vi "Consumer.vi"(8 "error in (no error)":errorcluster, 9 "Data":variant, 10 "Case ID":string, 11 "uService Template in":refnum<class "Common GUI v3.lvclass">) -> (0 "error out":errorcluster, 3 "uService Template out":refnum<class "Common GUI v3.lvclass">)   [LabVIEW 2026, in "TALOS.lvlib" / "Common GUI v3.lvlib" / "Common GUI v3.lvclass"]
uses:
  Common GUI v3.lvclass
  C:/LabVIEW Code/TALOS/talos/Ancestor/Ancestor/Ancestor.lvclass
  Common GUI v3 Consumer Case Selector.ctl
  Classes/Guardian List/Guardian List.lvclass
  Common GUI v3.lvclass/Common GUI v3.ctl
  Ancestor/Ancestor/Ancestor.lvclass/Ancestor.ctl
  Error Listbox Msg.ctl
  Error Listbox Msg Action.ctl
  Error Manager/Error Info.ctl
  Remote uService GUI.ctl
  Classes/uService List/uService List.lvclass/uService List.ctl
  Classes/uService List/Get Remote GUI.vi
  Classes/uService List/Get Remote Window VI Ref.vi
  Classes/uService List/Set Remote Window VI Ref.vi
  Classes/uService List/Get VI Ref.vi
  Support VIs/Generate Error.vi
  FGV/Error Memory/Get Error Description.vi
  Support VIs/Get PC name.vi
  Ancestor/Ancestor/Read ID.vi
  Support VIs/Get Class Name.vi
  FGV/Error Memory/Error Memory Core.vi
  <vilib>/AdvancedString/Delimited String to 1D String Array.vi
  <vilib>/AdvancedString/Delimited String to 1D String Array (string).vi
  Support VIs/Circus Root Path.vi
  FGV/Error Memory/Error Crt Lvl checker.vi
  FGV/Error Memory/Error Memory Core.vi/40c8088d-b597-4017-91af-faa98e00292e.vi
  FGV/Error Memory/Error Memory Core.vi/d4a3ab98-063c-4e44-b43d-fbdcfe6c2be2.vi
  Support VIs/Global Memory.vi
  <vilib>/Utility/LVClass/Get LV Class Name.vi
  Support VIs/Is in Packed Library.vi
  Support VIs/TALOS Root path.vi
  Support VIs/Read CSV worksheet.vi
  Support VIs/Global Constants.vi
  <vilib>/Utility/error.llb/General Error Handler.vi
  Support VIs/Error Log.vi
  Ancestor/Ancestor/Ancestor.lvclass
  <vilib>/Comparison/Equal/Equal Functor/Equal Functor.lvclass
  Classes/uService List/uService List.lvclass
  Father of all uServices/Father of all uServices/Father of all uServices.lvclass
  TALOS.lvlib
  Error Manager/Error Manager.lvclass
  Common GUI v3.lvlib
  Guardian/Guardian/Guardian.lvclass
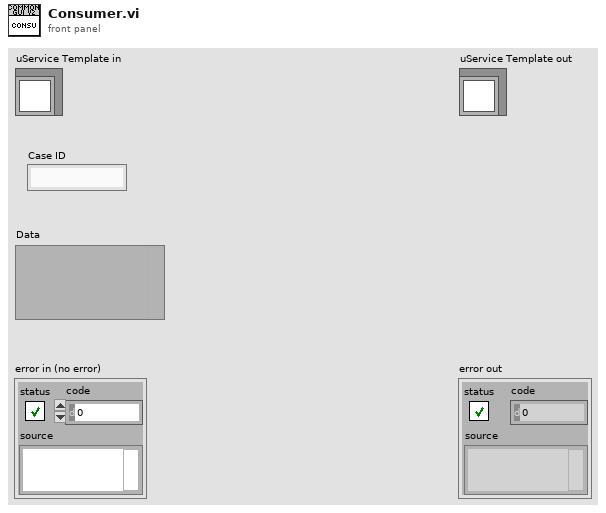
[diagram p1: front panel]
types:
  T1 = typedef "TALOS.lvlib/Common GUI v3.lvlib/Common GUI v3.lvclass/Common GUI v3 Consumer Case Selector.ctl" = enum16{"Update Guardians List", "Update ABORT LED", "Update Guardian ID", "Update Kasli Log", "Update Error Listbox", "Update Run Number", "Change Run LED color", "Update Run Status", "Run Stopped with Errors", "Reset Run LED", "Update Run Config", "Remote GUI"}
  T2 = typedef "TALOS.lvlib/Common GUI v3.lvlib/Common GUI v3.lvclass/Error Listbox Msg.ctl" = cluster{"Action":T3, "Error Info":T4}
  T3 = typedef "TALOS.lvlib/Common GUI v3.lvlib/Common GUI v3.lvclass/Error Listbox Msg Action.ctl" = enum16{"Add", "Remove", "Clear"}
  T4 = typedef "TALOS.lvlib/Error Manager.lvlib/Error Manager.lvclass/Error Info.ctl" = cluster{"error out":errorcluster, "Time Stamp":timestamp, "Machine Name":string, "GUID":string}
  T5 = typedef "TALOS.lvlib/Common GUI v3.lvlib/Remote uService GUI.ctl" = cluster{"Open/Close":bool, "uService ID":string}
  T6 = map{string, cluster{"Online":bool, "Last Poke":timestamp}}
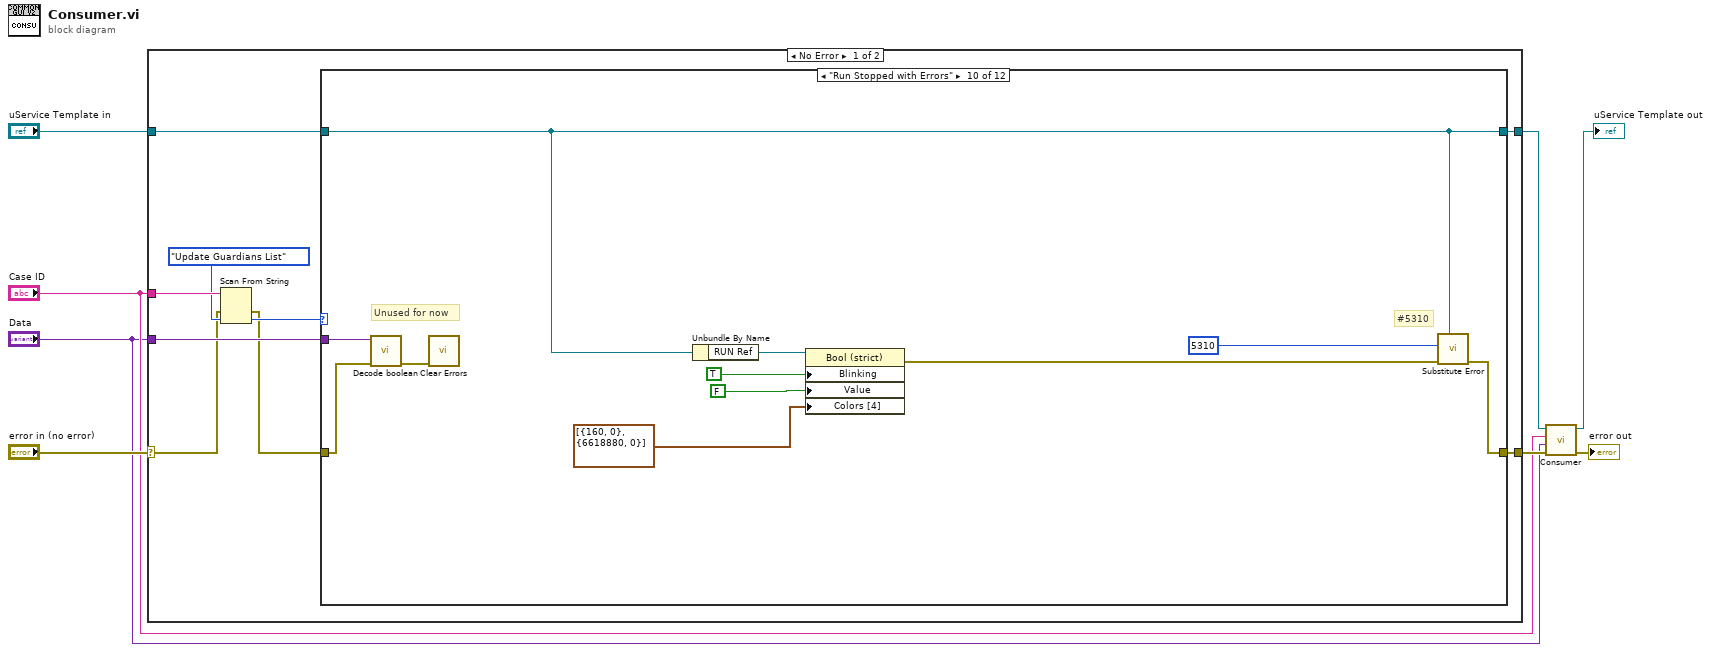
[diagram p0: block diagram]
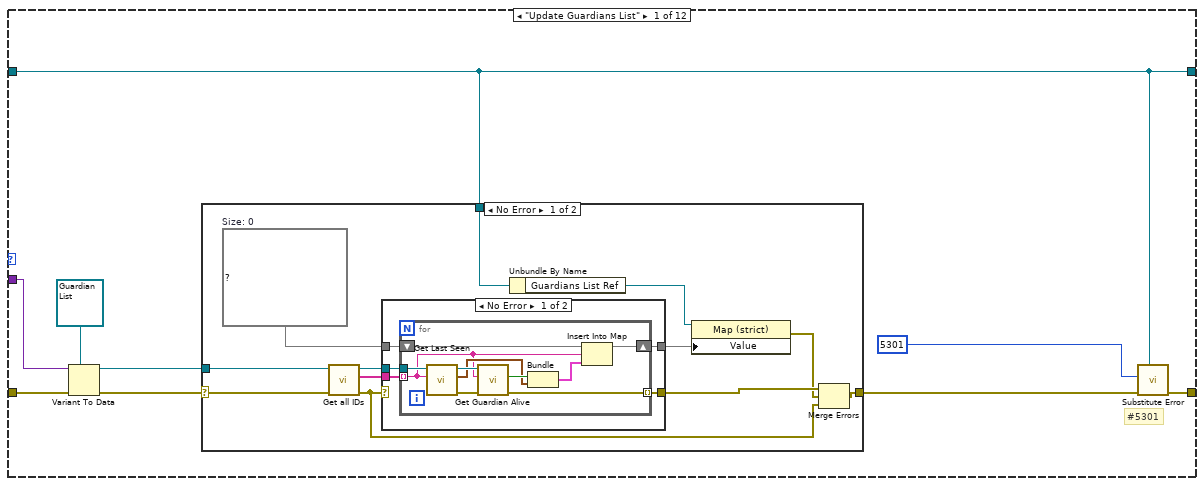
[diagram p2: hidden frame]
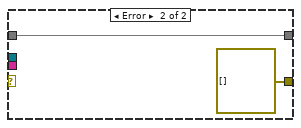
[diagram p3: hidden frame]
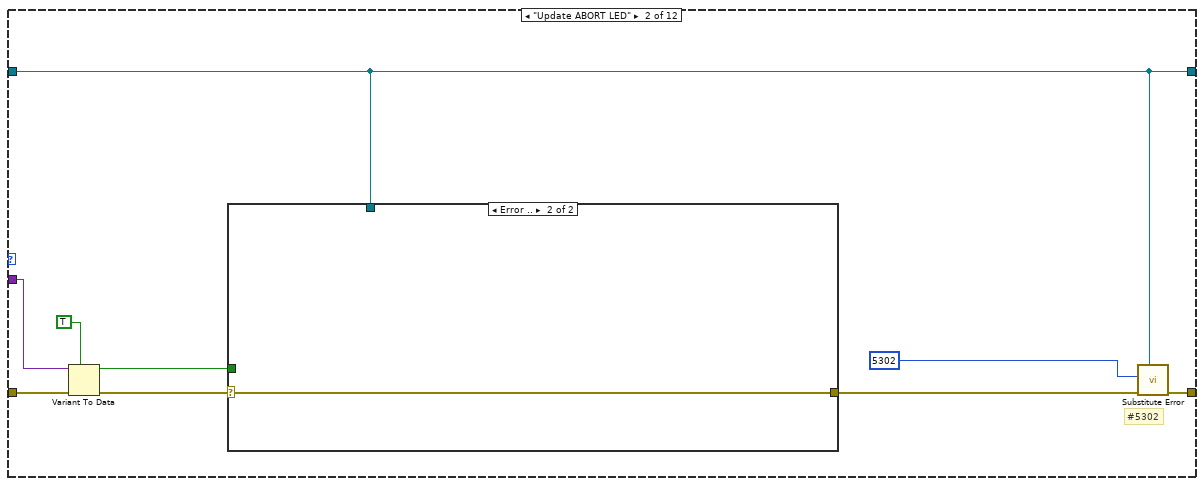
[diagram p5: hidden frame]
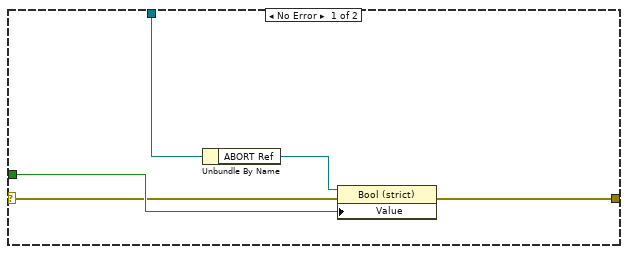
[diagram p6: hidden frame]
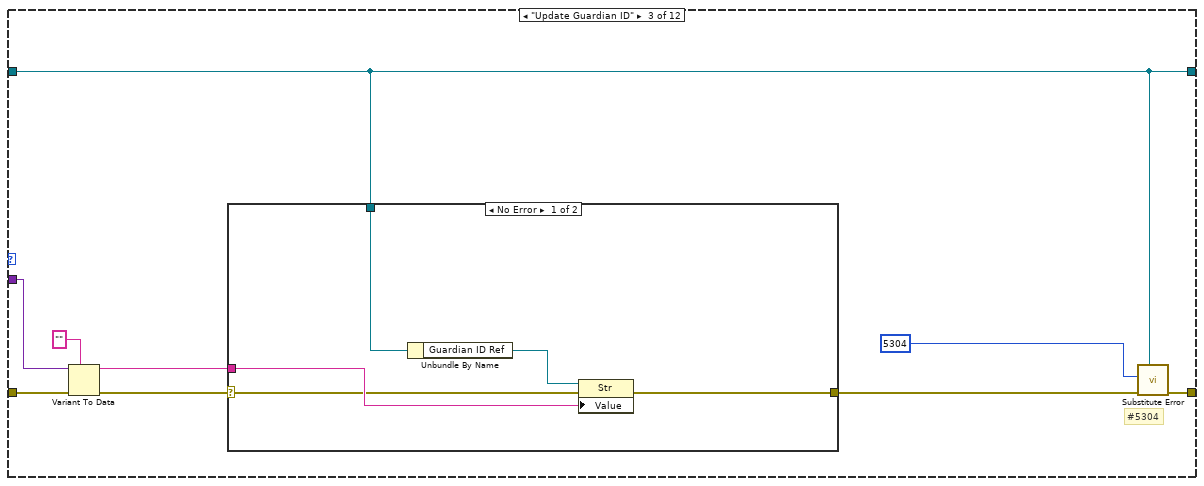
[diagram p7: hidden frame]
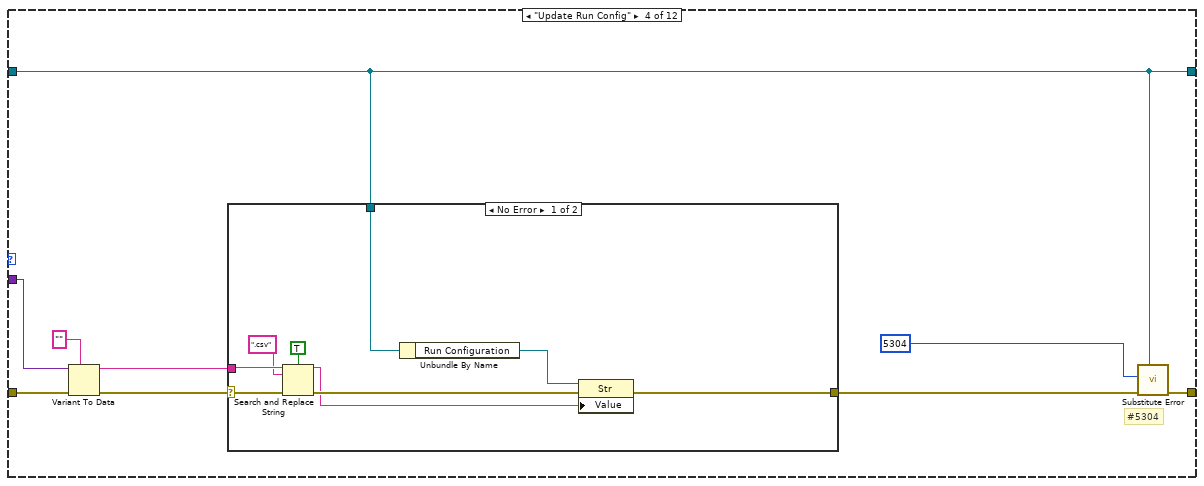
[diagram p9: hidden frame]
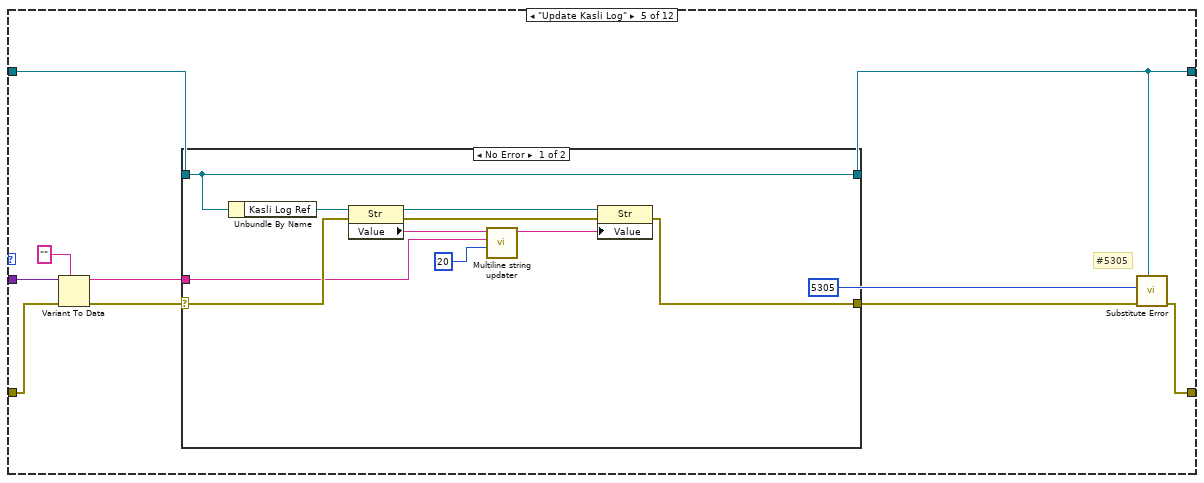
[diagram p11: hidden frame]
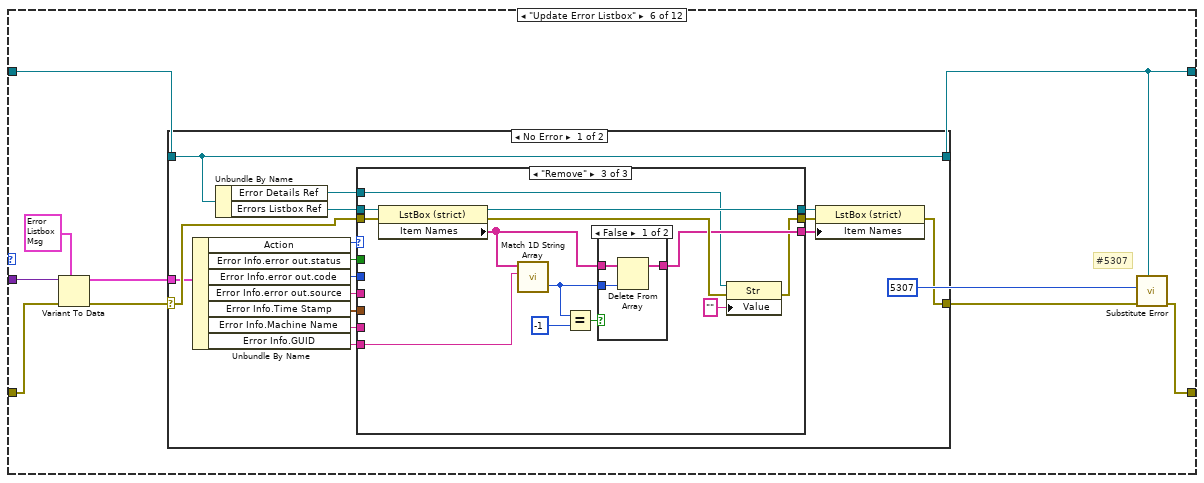
[diagram p13: hidden frame]
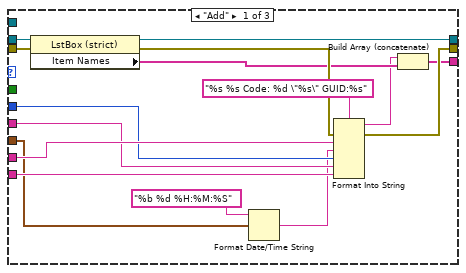
[diagram p14: hidden frame]
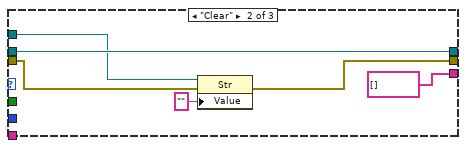
[diagram p15: hidden frame]
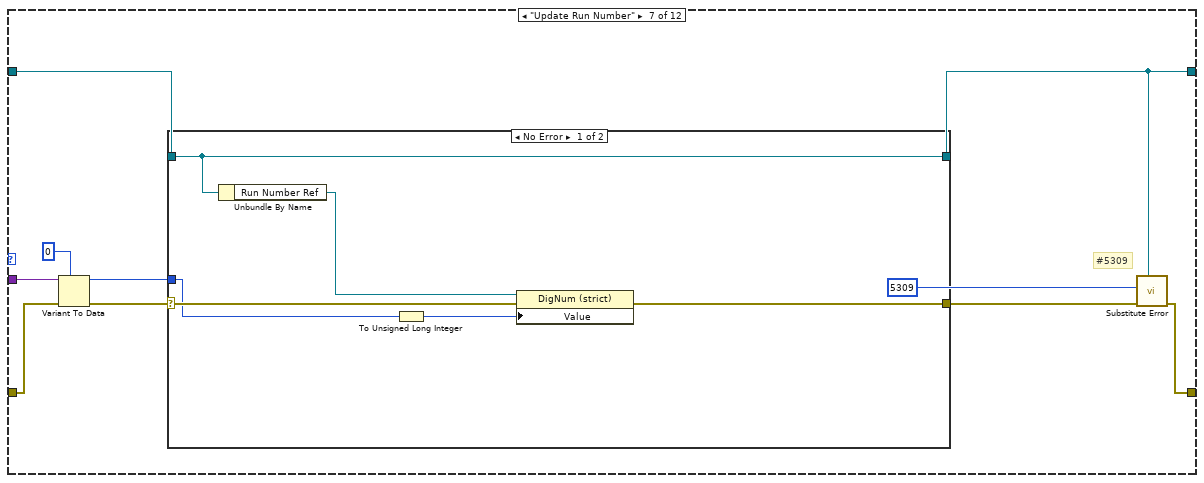
[diagram p18: hidden frame]
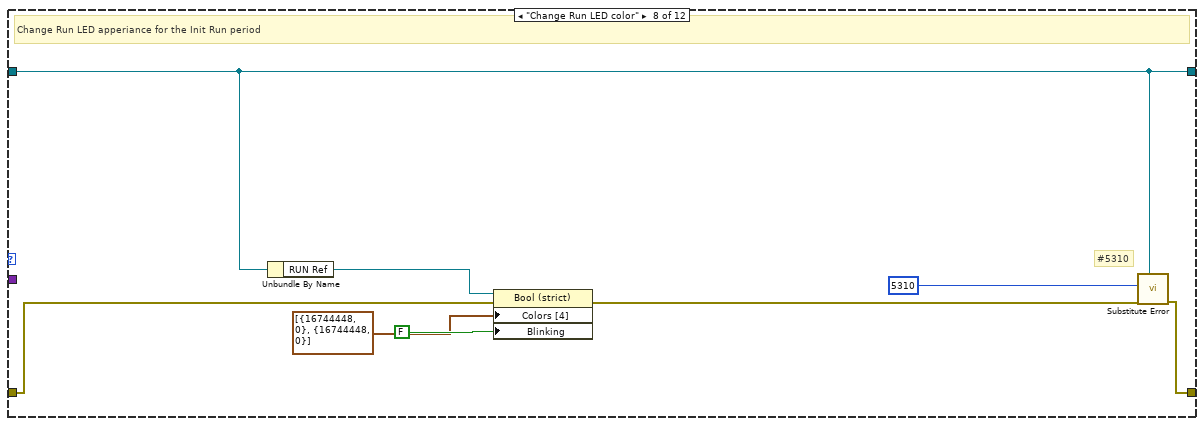
[diagram p20: hidden frame]
diagram:
  n1 = case shown="No Error" "error in (no error)" {
    selector: "error in (no error)" -> [w10 w352]
    tunnel: "uService Template in" -> [w16 w353]
    tunnel: [w14 w353] -> w4
    tunnel: [w15 w352] -> w3
    tunnel: "Case ID" -> [w13 _]
    tunnel: "Data" -> [w17 _]
    frame No Error {
      n2 = Scan From String(input string=w13, error in=w10, default 1=Common_GUI_v3_Consumer_Case_Selector."Update Guardians List") -> (error out=w9:errorcluster, output 1=w11:T1)  [unwired: 2 in, 2 out]
      n3 = case shown="\"Run Stopped with Errors\"" w11 {
        tunnel: w17 -> [w23 w63 w78 w93 w114 w136 w203 _ w225 w239 _ w260]
        tunnel: w9 -> [w22 w62 w77 w92 w112 w135 w202 w216 w224 w238 _ w259]
        tunnel: w16 -> [w19 w59 w74 w89 w115 w137 w204 w217 w226 w243 w249 w257]
        tunnel: [w20 w60 w75 w90 w109 w132 w199 w218 w227 w244 w250 w258] -> w15
        tunnel: [w19 w59 w74 w89 w108 w131 w198 w217 w226 w243 w249 w255] -> w14
        frame "Update Guardians List" {
          # "#5301"
          n4 = Variant To Data(error in=w22, type=refnum<class "Guardian List.lvclass"> refnum ("Guardian List in"), Variant=w23) -> (data=w24:refnum<class "Guardian List.lvclass">, error out=w26:errorcluster)
          n5 = case shown="No Error" w26 {
            selector: w26 -> [w35 w56]
            tunnel: w24 -> [w34 _]
            tunnel: w19 -> [w32 _]
            tunnel: [w29 w56] -> w21
            frame No Error {
              w36 = T6 {}  # Size: 0
              n6 = call-dynamic "Get all IDs.vi"("error in (no error)"=w35, "Guardian List in"=w34) -> ("error out"=w27:errorcluster, "All IDs"=w38:string[], "Guardian List out"=w37:refnum<class "Guardian List.lvclass">)  [unwired: 7 in]
              n7 = case shown="No Error" w27 {
                tunnel: w38 -> [w43 _]
                tunnel: w37 -> [w42 _]
                tunnel: w36 -> [w41 w55]
                tunnel: [w40 errorcluster[] []] -> w33
                tunnel: [w39 w55] -> w30
                frame No Error {
                  n8 = for {
                    tunnel: w43 -> [w47] mode=indexing
                    tunnel: w42 -> [w53]
                    shift-right: [w48] -> w39
                    shift-left: w41 -> [w49]
                    tunnel: [w45] -> w40 mode=indexing
                    n9 = call-dynamic "Get Last Seen.vi"("ID"=w47, "Guardian List in"=w53) -> ("error out"=w44:errorcluster, "Last Poke"=w50:timestamp, "Guardian List out"=w52:refnum<class "Guardian List.lvclass">)  [unwired: 7 in]
                    n10 = call-dynamic "Get Guardian Alive.vi"("error in (no error)"=w44, "ID"=w47, "Guardian List in"=w52) -> ("error out"=w45:errorcluster, "Alive"=w51:bool)  [unwired: 6 in, 1 out]
                    n11 = Bundle("Alive"=w51, "Last Poke"=w50) -> (w46:cluster{"Alive":bool, "Last Poke":timestamp})  [unwired: 1 in]
                    n12 = Insert Into Map(map in=w49, key=w47, value=w46) -> (map out=w48:T6)  [unwired: 2 out]
                  }
                }
                frame Error {
                }
              }
              n13 = Unbundle By Name(w32) -> ("Guardians List Ref"=w31:refnum<vi>)
              n14 = property class="Map (strict)"(reference=w31, "Value"=w30) -> (error out=w28:errorcluster)  [unwired: 1 in, 1 out]
              n15 = Merge Errors(w33, w28, w27) -> (w29:errorcluster)
            }
            frame Error {
            }
          }
          n16 = call "Substitute Error.vi"("LabVIEW Object"=w19, "error in (no error)"=w21, "Error Code"=5301) -> ("error out"=w20:errorcluster)  [unwired: 8 in]
        }
        frame "Update ABORT LED" {
          # "#5302"
          n17 = Variant To Data(error in=w62, type=TRUE, Variant=w63) -> (data=w64:bool, error out=w65:errorcluster)
          n18 = case shown="Error .." w65 {
            selector: w65 -> [w67 w71]
            tunnel: w64 -> [w68 _]
            tunnel: w59 -> [w70 _]
            tunnel: [w69 w71] -> w61
            frame No Error {
              n19 = Unbundle By Name(w70) -> ("ABORT Ref"=w66:refnum<vi>)
              n20 = property class="Bool (strict)"(reference=w66, error in=w67, "Value"=w68) -> (error out=w69:errorcluster)  [unwired: 1 out]
            }
            frame Error {
            }
          }
          n21 = call "Substitute Error.vi"("LabVIEW Object"=w59, "error in (no error)"=w61, "Error Code"=5302) -> ("error out"=w60:errorcluster)  [unwired: 8 in]
        }
        frame "Update Guardian ID" {
          # "#5304"
          n22 = Variant To Data(error in=w77, type="", Variant=w78) -> (data=w79:string, error out=w80:errorcluster)
          n23 = case shown="No Error" w80 {
            selector: w80 -> [w82 w86]
            tunnel: w79 -> [w83 _]
            tunnel: w74 -> [w85 _]
            tunnel: [w84 w86] -> w76
            frame No Error {
              n24 = Unbundle By Name(w85) -> ("Guardian ID Ref"=w81:refnum<vi>)
              n25 = property class="Str"(reference=w81, error in=w82, "Value"=w83) -> (error out=w84:errorcluster)  [unwired: 1 out]
            }
            frame Error {
            }
          }
          n26 = call "Substitute Error.vi"("LabVIEW Object"=w74, "error in (no error)"=w76, "Error Code"=5304) -> ("error out"=w75:errorcluster)  [unwired: 8 in]
        }
        frame "Update Run Config" {
          # "#5304"
          n27 = Variant To Data(error in=w92, type="", Variant=w93) -> (data=w94:string, error out=w95:errorcluster)
          n28 = case shown="No Error" w95 {
            selector: w95 -> [w101 w105]
            tunnel: w94 -> [w99 _]
            tunnel: w89 -> [w104 _]
            tunnel: [w103 w105] -> w91
            frame No Error {
              n29 = Search and Replace String(case sensitive?=TRUE ("ignore case? (F)"), input string=w99, search string=".csv", error in=w101) -> (result string=w96:string, error out=w100:errorcluster)  [unwired: 4 in, 2 out]
              n30 = Unbundle By Name(w104) -> ("Run Configuration"=w102:refnum<vi>)
              n31 = property class="Str"(reference=w102, error in=w100, "Value"=w96) -> (error out=w103:errorcluster)  [unwired: 1 out]
            }
            frame Error {
            }
          }
          n32 = call "Substitute Error.vi"("LabVIEW Object"=w89, "error in (no error)"=w91, "Error Code"=5304) -> ("error out"=w90:errorcluster)  [unwired: 8 in]
        }
        frame "Update Kasli Log" {
          # "#5305"
          n33 = Variant To Data(error in=w112, type="", Variant=w114) -> (data=w106:string, error out=w111:errorcluster)
          n34 = case shown="No Error" w111 {
            selector: w111 -> [w124 w126]
            tunnel: w115 -> [w116 w127]
            tunnel: [w116 w127] -> w108
            tunnel: [w117 w126] -> w110
            tunnel: w106 -> [w119 _]
            frame No Error {
              n35 = Unbundle By Name(w116) -> ("Kasli Log Ref"=w125:refnum<vi>)
              n36 = property class="Str"(reference=w125, error in=w124) -> (reference out=w123:refnum<vi>, error out=w122:errorcluster, "Value"=w121:string)
              n37 = call "Multiline string updater.vi"("Lines to keep"=u8 20, "String to add"=w119, "Multiline string in"=w121) -> ("Multiline string out"=w120:string)  [unwired: 8 in]
              n38 = property class="Str"(reference=w123, error in=w122, "Value"=w120) -> (error out=w117:errorcluster)  [unwired: 1 out]
            }
            frame Error {
            }
          }
          n39 = call "Substitute Error.vi"("LabVIEW Object"=w108, "error in (no error)"=w110, "Error Code"=5305) -> ("error out"=w109:errorcluster)  [unwired: 8 in]
        }
        frame "Update Error Listbox" {
          # "#5307"
          n40 = Variant To Data(error in=w135, type=T2 {"Action"=enum."Add", "Error Info"={"error out"={"status"=FALSE, "code"=0, "source"=""}, "Time Stamp"=timestamp(0 s since 1904-01-01), "Machine Name"="", "GUID"=""}} ("Error Listbox Msg"), Variant=w136) -> (data=w129:T2, error out=w134:errorcluster)
          n41 = case shown="No Error" w134 {
            selector: w134 -> [w152 w193]
            tunnel: w137 -> [w151 w194]
            tunnel: [w151 w194] -> w131
            tunnel: [w139 w193] -> w133
            tunnel: w129 -> [w150 _]
            frame No Error {
              n42 = Unbundle By Name(w150) -> ("Action"=w149:T3, "Error Info.error out.status"=w148:bool, "Error Info.error out.code"=w147:i32, "Error Info.error out.source"=w146:string, "Error Info.Time Stamp"=w145:timestamp, "Error Info.Machine Name"=w144:string, "Error Info.GUID"=w143:string)
              n43 = Unbundle By Name(w151) -> ("Error Details Ref"=w138:refnum<vi>, "Errors Listbox Ref"=w153:refnum<vi>)
              n44 = case shown="\"Remove\"" w149 {
                tunnel: w153 -> [w169 w175 w187]
                tunnel: w152 -> [w168 w172 w186]
                tunnel: w148 -> [_ _ _]
                tunnel: w147 -> [w162 _ _]
                tunnel: w146 -> [w161 _ _]
                tunnel: w145 -> [w155 _ _]
                tunnel: w144 -> [w164 _ _]
                tunnel: w143 -> [w160 _ w182]
                tunnel: [w159 w175 w185] -> w142
                tunnel: [w158 w171 w176] -> w141
                tunnel: [w157 string[] [] ("Item Names") w184] -> w140
                tunnel: w138 -> [_ w173 w177]
                frame "Add" {
                  n45 = property class="LstBox (strict)"(reference=w169, error in=w168) -> (reference out=w159:refnum<vi>, error out=w167:errorcluster, "Item Names"=w166:string[])
                  n46 = Format Date/Time String(time format string (%c)="%b %d %H:%M:%S", seconds (now)=w155) -> (date/time string=w154:string)  [unwired: 1 in]
                  n47 = Format Into String(format string="%s %s Code: %d \"%s\" GUID:%s", error in=w167, w164, w154, w162, w161, w160) -> (resulting string=w165:string, error out=w158:errorcluster)  [unwired: 1 in]
                  n48 = Build Array (concatenate)(w165, w166) -> (w157:string[])
                }
                frame "Clear" {
                  n49 = property class="Str"(reference=w173, error in=w172, "Value"="") -> (error out=w171:errorcluster)  [unwired: 1 out]
                }
                frame "Remove" {
                  n50 = property class="LstBox (strict)"(reference=w187, error in=w186) -> (reference out=w185:refnum<vi>, error out=w188:errorcluster, "Item Names"=w183:string[])
                  n51 = call <vilib>:"Match 1D String Array.vi"("Pattern"=w182, "Strings"=w183) -> ("index of element"=w180:i32)  [unwired: 2 in, 1 out]
                  n52 = Equal?(x=w180, y=-1) -> (x = y?=w179:bool)
                  n53 = case shown="False" w179 {
                    tunnel: [w191 w192] -> w184
                    tunnel: w183 -> [w190 w192]
                    tunnel: w180 -> [w189 _]
                    frame False {
                      n54 = Delete From Array(array=w190, index=w189) -> (array with subset deleted=w191:string[])  [unwired: 1 in, 1 out]
                    }
                    frame True {
                      # "Not found!"
                    }
                  }
                  n55 = property class="Str"(reference=w177, error in=w188, "Value"="") -> (error out=w176:errorcluster)  [unwired: 1 out]
                }
              }
              n56 = property class="LstBox (strict)"(reference=w142, error in=w141, "Item Names"=w140) -> (error out=w139:errorcluster)  [unwired: 1 out]
            }
            frame Error {
            }
          }
          n57 = call "Substitute Error.vi"("LabVIEW Object"=w131, "error in (no error)"=w133, "Error Code"=5307) -> ("error out"=w132:errorcluster)  [unwired: 8 in]
        }
        frame "Update Run Number" {
          # "#5309"
          n58 = Variant To Data(error in=w202, type=0, Variant=w203) -> (data=w196:i32, error out=w201:errorcluster)
          n59 = case shown="No Error" w201 {
            selector: w201 -> [w207 w211]
            tunnel: w204 -> [w210 w212]
            tunnel: [w210 w212] -> w198
            tunnel: [w209 w211] -> w200
            tunnel: w196 -> [w205 _]
            frame No Error {
              n60 = Unbundle By Name(w210) -> ("Run Number Ref"=w208:refnum<vi>)
              n61 = To Unsigned Long Integer(number=w205) -> (unsigned 32bit integer=w206:u32)
              n62 = property class="DigNum (strict)"(reference=w208, error in=w207, "Value"=w206) -> (error out=w209:errorcluster)  [unwired: 1 out]
            }
            frame Error {
            }
          }
          n63 = call "Substitute Error.vi"("LabVIEW Object"=w198, "error in (no error)"=w200, "Error Code"=5309) -> ("error out"=w199:errorcluster)  [unwired: 8 in]
        }
        frame "Change Run LED color" {
          # "#5310"
          # "Change Run LED apperiance for the Init Run period"
          n64 = Unbundle By Name(w217) -> ("RUN Ref"=w214:refnum<vi>)
          n65 = property class="Bool (strict)"(reference=w214, error in=w216, "Colors [4]"=cluster{u32, u32}[] [{16744448, 0}, {16744448, 0}], "Blinking"=FALSE) -> (error out=w219:errorcluster)  [unwired: 1 out]
          n66 = call "Substitute Error.vi"("LabVIEW Object"=w217, "error in (no error)"=w219, "Error Code"=5310) -> ("error out"=w218:errorcluster)  [unwired: 8 in]
        }
        frame "Update Run Status" {
          # "#5310"
          n67 = Variant To Data(error in=w224, type=TRUE, Variant=w225) -> (data=w221:bool, error out=w223:errorcluster)
          n68 = case shown="No Error" w223 {
            selector: w223 -> [w232 w236]
            tunnel: [w235 w236] -> w229
            tunnel: w226 -> [w233 _]
            tunnel: w221 -> [w231 _]
            frame No Error {
              n69 = Unbundle By Name(w233) -> ("RUN Ref"=w234:refnum<vi>)
              n70 = property class="Bool (strict)"(reference=w234, error in=w232, "Value"=w231, "Colors [4]"=cluster{u32, u32}[] [{160, 0}, {6618880, 0}]) -> (error out=w235:errorcluster)  [unwired: 1 out]
            }
            frame Error {
            }
          }
          n71 = call "Substitute Error.vi"("LabVIEW Object"=w226, "error in (no error)"=w229, "Error Code"=5310) -> ("error out"=w227:errorcluster)  [unwired: 8 in]
        }
        frame "Run Stopped with Errors" {
          # "Unused for now"
          # "#5310"
          n72 = call "Decode boolean.vi"("error in (no error)"=w238, "Data"=w239) -> ("error out"=w237:errorcluster)  [unwired: 8 in, 1 out]
          n73 = call <vilib>:"Clear Errors.vi"("error in (no error)"=w237) -> ()  [unwired: 5 in, 2 out]
          n74 = Unbundle By Name(w243) -> ("RUN Ref"=w247:refnum<vi>)
          n75 = property class="Bool (strict)"(reference=w247, "Blinking"=TRUE, "Value"=FALSE, "Colors [4]"=cluster{u32, u32}[] [{160, 0}, {6618880, 0}] ("Colors")) -> (error out=w245:errorcluster)  [unwired: 1 in, 1 out]
          n76 = call "Substitute Error.vi"("LabVIEW Object"=w243, "error in (no error)"=w245, "Error Code"=5310) -> ("error out"=w244:errorcluster)  [unwired: 8 in]
        }
        frame "Reset Run LED" {
          # "#5310"
          n77 = Unbundle By Name(w249) -> ("RUN Ref"=w254:refnum<vi>)
          n78 = property class="Bool (strict)"(reference=w254, "Blinking"=FALSE, "Colors [4]"=cluster{u32, u32}[] [{160, 0}, {6618880, 0}] ("Colors")) -> (error out=w251:errorcluster)  [unwired: 1 in, 1 out]
          n79 = call "Substitute Error.vi"("LabVIEW Object"=w249, "error in (no error)"=w251, "Error Code"=5310) -> ("error out"=w250:errorcluster)  [unwired: 8 in]
        }
        frame "Remote GUI" {
          n80 = property class="Common GUI v3.lvclass"(reference=w257) -> (reference out=w255:refnum<class "Common GUI v3.lvclass">, "Accessors:uS List Ref"=w256:refnum<data-value>)  [unwired: 1 in, 1 out]
          n81 = Variant To Data(error in=w259, type=T5 {"Open/Close"=FALSE, "uService ID"=""} ("Remote GUI"), Variant=w260) -> (data=w261:T5, error out=w262:errorcluster)
          n82 = case shown="No Error" w262 {
            selector: w262 -> [_ w351]
            tunnel: w261 -> [w270 _]
            tunnel: [w269 w350] -> w258
            tunnel: w255 -> [w266 w348]
            tunnel: w256 -> [w265 _]
            tunnel: w255 -> [w264 _]
            frame No Error {
              n83 = in-place {
                in-place-border: w270 -> [w282]
                in-place-border: [w276] -> w268
                in-place-border: [w275] -> w267
                in-place-border: w264 -> [w272]
                n84 = in-place-dvr #1(w265) -> (w274:refnum<class "uService List.lvclass">, w273:errorcluster)
                n85 = Unbundle(w282) -> ("Open/Close"=w281:bool, "uService ID"=w278:string)
                n86 = call-poly "uService List.vi"("error in (no error)"=w273, "ID"=w278, "uService List in"=w274) -> ("error out"=w277:errorcluster, "Remote GUI"=w279:bool, "uService List out"=w280:refnum<class "uService List.lvclass">)  [unwired: 6 in]
                n87 = case shown="False" w281 {
                  tunnel: w280 -> [w294 w323]
                  tunnel: w279 -> [w295 w324]
                  tunnel: w278 -> [w292 w322]
                  tunnel: w277 -> [w293 w321]
                  tunnel: [w290 w320] -> w276
                  tunnel: w272 -> [w284 w319]
                  tunnel: [w291 w318] -> w275
                  tunnel: [w283 w317] -> w271
                  frame False {
                    w291 = 5316  # #5316
                    # "Close remote window"
                    n88 = case shown="False" w295 {
                      tunnel: w294 -> [w296 w310]
                      tunnel: w293 -> [w297 w309]
                      tunnel: w292 -> [_ w306]
                      tunnel: [w297 w299] -> w289
                      tunnel: [w296 w298] -> w283
                      frame False {
                        # "already closed, do noting"
                      }
                      frame True {
                        n89 = call-poly "uService List.vi"("error in (no error)"=w309, "ID"=w306, "uService List in"=w310) -> ("error out"=w305:errorcluster, "Vi Ref"=w307:refnum<vi>, "uService List out"=w308:refnum<class "uService List.lvclass">)  [unwired: 6 in]
                        n90 = call "Close Remote uService GUI.vi"("error in (no error)"=w305, "Remote GUI"=w307) -> ("error out"=w304:errorcluster, "reference out"=w303:refnum<vi>)  [unwired: 8 in]
                        n91 = case shown="No Error" w304 {
                          selector: w304 -> [w311 w313]
                          tunnel: w303 -> [_ w316]
                          tunnel: [w311 w312] -> w300
                          frame No Error {
                          }
                          frame Error {
                            n92 = invoke class="VI" method="Abort VI"(reference=w316, error in=w313) -> (reference out=w315:refnum<vi>, error out=w314:errorcluster)  [unwired: 1 in, 1 out]
                            n93 = invoke class="VI" method="FP.Close"(reference=w315, error in=w314) -> (error out=w312:errorcluster)  [unwired: 1 in, 2 out]
                          }
                        }
                        n94 = call-poly "uService List.vi"("Vi Ref"=refnum<vi> refnum, "ID"=w306, "uService List in"=w308) -> ("error out"=w301:errorcluster, "uService List out"=w298:refnum<class "uService List.lvclass">)  [unwired: 7 in]
                        n95 = Merge Errors(w301, w300) -> (w299:errorcluster)
                      }
                    }
                    n96 = Unbundle By Name(w284) -> ("uService to show"=w286:refnum<vi>)
                    n97 = property class="CmbBox"(reference=w286, error in=w289) -> (reference out=w285:refnum<vi>, error out=w287:errorcluster, "Value"=w288:string)
                    n98 = property class="CmbBox"(reference=w285, error in=w287, "Val(Sgnl)"=w288) -> (error out=w290:errorcluster)  [unwired: 1 out]
                  }
                  frame True {
                    w318 = 5315  # #5315
                    # "Open remote window"
                    n99 = case shown="False" w324 {
                      tunnel: w323 -> [w330 w346]
                      tunnel: w322 -> [w328 w342]
                      tunnel: w321 -> [w329 w347]
                      tunnel: [w334 w341] -> w320
                      tunnel: w319 -> [w333 _]
                      tunnel: [w325 w340] -> w317
                      frame False {
                        n100 = Unbundle By Name(w333) -> ("Sub Panel Reference"=w332:refnum<vi>)
                        n101 = call-poly "uService List.vi"("error in (no error)"=w329, "ID"=w328, "uService List in"=w330) -> ("error out"=w339:errorcluster, "Vi Ref"=w327:refnum<vi>, "uService List out"=w326:refnum<class "uService List.lvclass">)  [unwired: 6 in]
                        n102 = invoke class="SubPnl" method="Remove VI"(reference=w332, error in=w339) -> (error out=w331:errorcluster)  [unwired: 1 in, 2 out]
                        n103 = call "Open Remote uService GUI.vi"("error in (no error)"=w331, "GUI VI"=w327, "uService ID"=w328, "Message Enqueuer"=w333) -> ("error out"=w336:errorcluster, "Remote GUI ref"=w338:refnum<vi>, "uService ID dup"=w335:string)  [unwired: 5 in]
                        n104 = call-poly "uService List.vi"("Vi Ref"=w338, "ID"=w335, "uService List in"=w326) -> ("error out"=w337:errorcluster, "uService List out"=w325:refnum<class "uService List.lvclass">)  [unwired: 7 in]
                        n105 = Merge Errors(w337, w336) -> (w334:errorcluster)
                      }
                      frame True {
                        n106 = call-poly "uService List.vi"("error in (no error)"=w347, "ID"=w342, "uService List in"=w346) -> ("error out"=w344:errorcluster, "Vi Ref"=w345:refnum<vi>, "uService List out"=w340:refnum<class "uService List.lvclass">)  [unwired: 6 in]
                        n107 = property class="VI"(reference=w345, error in=w344, "Front Panel.IsFrontmost"=TRUE ("Front Panel Window:Is Frontmost")) -> (error out=w341:errorcluster)  [unwired: 1 out]
                      }
                    }
                  }
                }
                n108 = in-place-dvr #1(w271) -> ()  [unwired: 2 out]
              }
              n109 = call "Substitute Error.vi"("LabVIEW Object"=w266, "error in (no error)"=w268, "Error Code"=w267) -> ("error out"=w269:errorcluster)  [unwired: 8 in]
            }
            frame Error {
              w349 = 5317  # #5317
              n110 = call "Substitute Error.vi"("LabVIEW Object"=w348, "error in (no error)"=w351, "Error Code"=w349) -> ("error out"=w350:errorcluster)  [unwired: 8 in]
            }
          }
        }
      }
    }
    frame Error {
    }
  }
  n111 = call-parent "Consumer.vi"("error in (no error)"=w3, "Data"="Data", "Case ID"="Case ID", "uService Template in"=w4) -> ("error out"=→"error out":errorcluster, "uService Template out"=→"uService Template out":refnum<class "Common GUI v3.lvclass">)  [unwired: 6 in]
